vi "Read INI String.vi"(6 "Force Default Session?(F)":bool, 8 "error in (no error)":errorcluster, 9 "Default":string, 10 "Variable":T1, 11 "CSM-Static-Variable-Manager in":refnum<class "CSM-Static-Variable-Manager.lvclass">) -> (0 "error out":errorcluster, 1 "Content":string, 2 "Key Found?":bool, 3 "CSM-Static-Variable-Manager out":refnum<class "CSM-Static-Variable-Manager.lvclass">, 5 "Section Name":string)   [LabVIEW 2017, in "INI-Static-Variable-Support.lvlib" / "CSM-Static-Variable-Manager.lvclass"]
uses:
  CSM-Static-Variable-Manager.lvclass
  _Def-Ini-Variable.ctl
  CSM-Static-Variable-Manager.lvclass/CSM-Static-Variable-Manager.ctl
  INI-Static-Variable-Support.lvlib
  LabVIEW-Config/LabVIEW-Config.lvlib
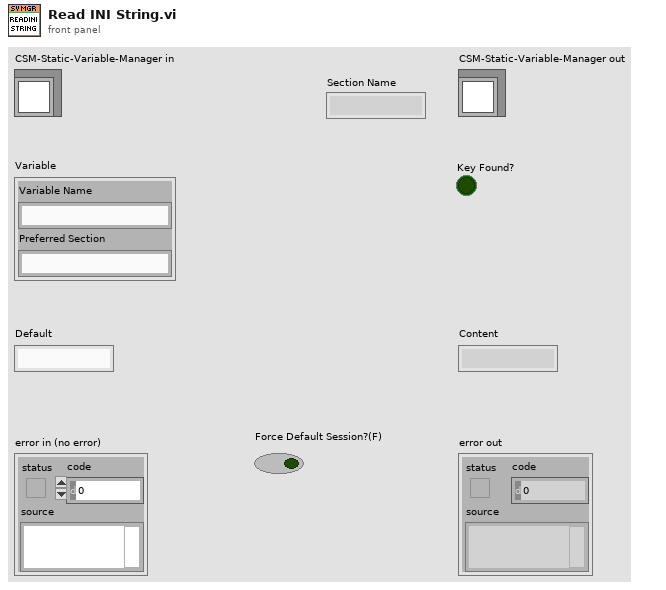
[diagram p1: front panel]
types:
  T1 = typedef "INI-Static-Variable-Support.lvlib/_Def-Ini-Variable.ctl" = cluster{"Variable Name":string, "Preferred Section":string}
  T2 = typedef "LabVIEW-Config.lvlib/Config.ctl" = cluster{"Path":path, "Lines":string[], "Tokens":T3[], "Modified?":bool}
  T3 = typedef "LabVIEW-Config.lvlib/LineToken.ctl" = enum8{"comment", "section", "key", "more"}
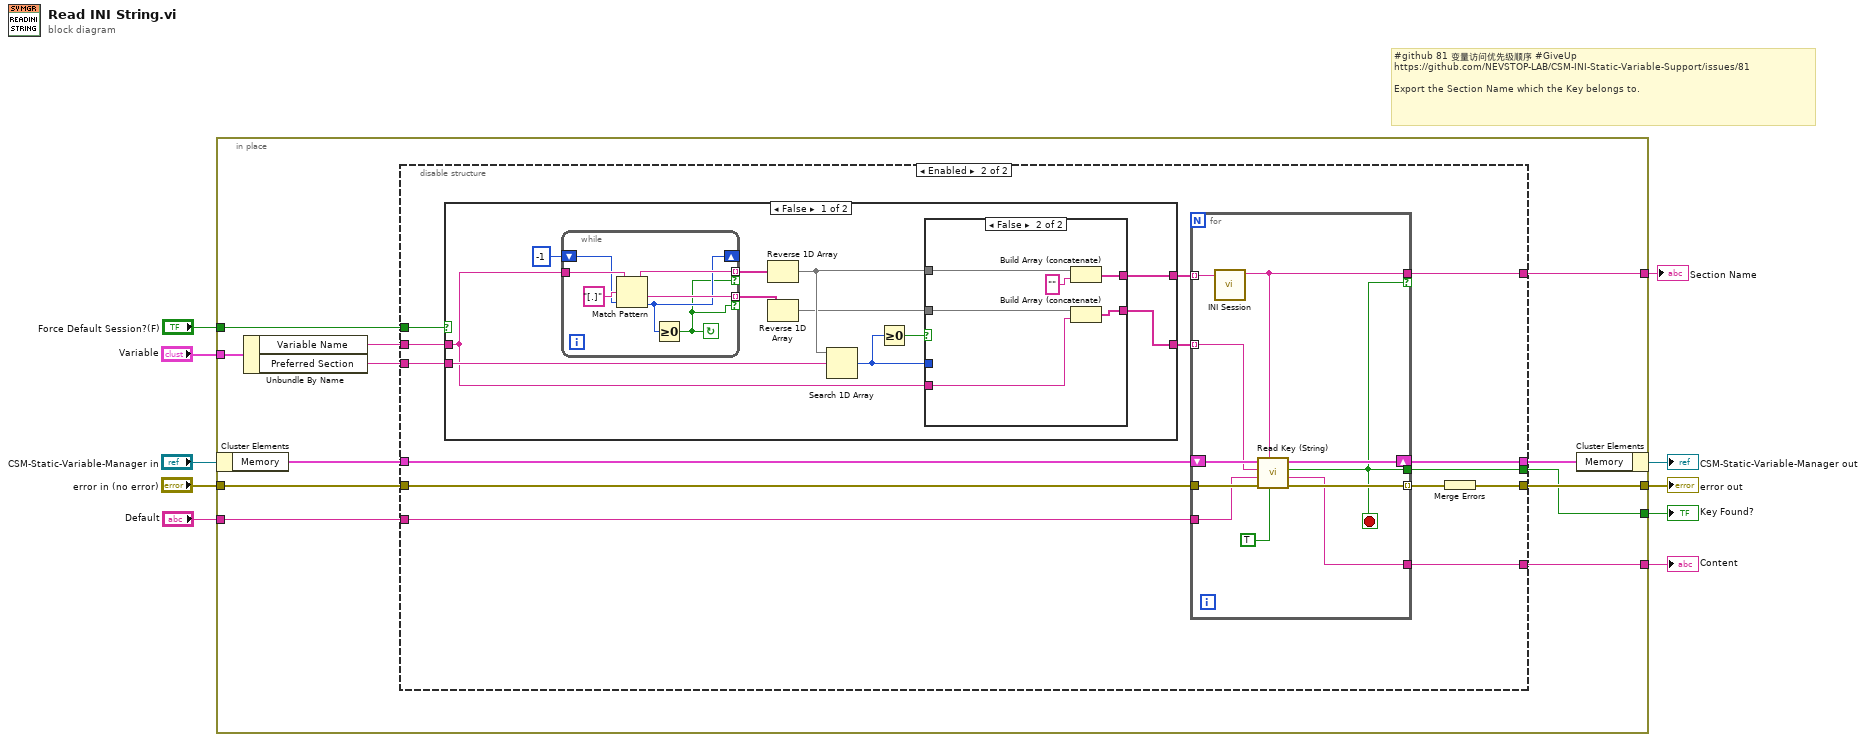
[diagram p0: block diagram]
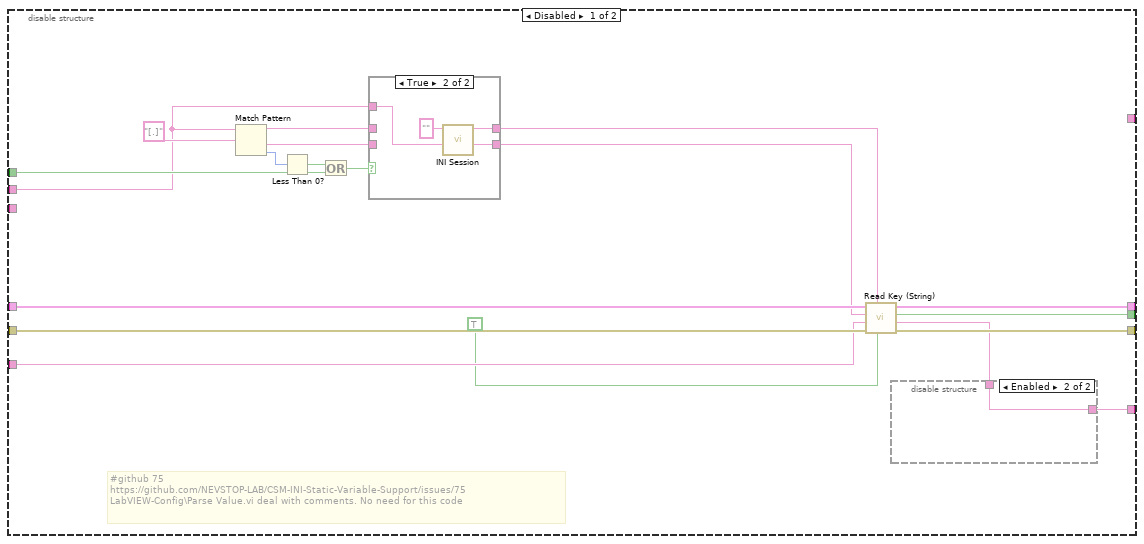
[diagram p2: hidden frame]
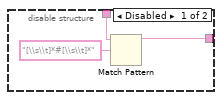
[diagram p3: hidden frame]
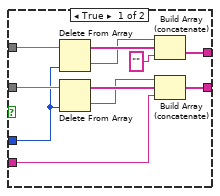
[diagram p5: hidden frame]
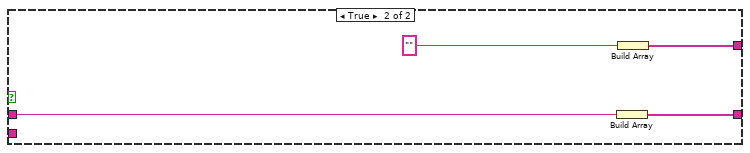
[diagram p6: hidden frame]
diagram:
  # "#github 81 变量访问优先级顺序 #GiveUp\nhttps://github.com/NEVSTOP-LAB/CSM-INI-Static-Variable-Support/issues/81\n\nExport the Section Name which the Key belongs to."
  n1 = in-place {
    in-place-border: "error in (no error)" -> [w20]
    in-place-border: [w19] -> w7
    in-place-border: [w18] -> w6
    in-place-border: "Variable" -> [w16]
    in-place-border: "Force Default Session?(F)" -> [w17]
    in-place-border: [w14] -> w3
    in-place-border: "Default" -> [w15]
    in-place-border: [w11] -> w1
    n2 = in-place-cluster #1("CSM-Static-Variable-Manager in") -> ("Memory"=w22:T2)
    n3 = Unbundle By Name(w16) -> ("Variable Name"=w13:string, "Preferred Section"=w12:string)
    n4 = disable-structure shown="Enabled" {
      disable-tunnel: w22 -> [w41 w64]
      disable-tunnel: [w40 w63] -> w21
      disable-tunnel: w20 -> [w39 w62]
      disable-tunnel: [w38 w53] -> w19
      disable-tunnel: [w37 w60] -> w18
      disable-tunnel: w17 -> [w33 w59]
      disable-tunnel: w15 -> [w27 w56]
      disable-tunnel: [w25 w55] -> w14
      disable-tunnel: w13 -> [w23 w54]
      disable-tunnel: w12 -> [_ w52]
      disable-tunnel: [_ w51] -> w11
      frame Disabled {
        # "#github 75\nhttps://github.com/NEVSTOP-LAB/CSM-INI-Static-Variable-Support/issues/75 \nLabVIEW-Config\\Parse Value.vi deal with comments. No need for this code"
        n5 = Match Pattern(string=w23, regular expression="[.]") -> (before substring=w30:string, after substring=w29:string, offset past match=w35:i32)  [unwired: 1 in, 1 out]
        n6 = Less Than 0?(x=w35) -> (x < 0?=w34:bool)
        n7 = Or(x=w34, y=w33) -> (x .or. y?=w32:bool)
        n8 = case shown="True" w32 {
          tunnel: [w47 w50] -> w31
          tunnel: w30 -> [w47 _]
          tunnel: w23 -> [_ w49]
          tunnel: w29 -> [w46 _]
          tunnel: [w46 w49] -> w28
          frame False {
          }
          frame True {
            n9 = call "INI Session.vi"("Section Name(\"\" as Default)"="" ("Section Name(\"\" as Default)")) -> ("App.Name"=w50:string)  [unwired: 10 in]
          }
        }
        n10 = call "Read Key (String).vi"("Read Raw String? (F)"=TRUE, "Section Name"=w31, "error in (no error)"=w39, "Default"=w27, "Key Name"=w28, "Config in"=w41) -> ("error out"=w38:errorcluster, "Value"=w26:string, "Key Found?"=w37:bool, "Config out"=w40:T2)  [unwired: 2 in]
        n11 = disable-structure shown="Enabled" {
          disable-tunnel: w26 -> [w44 w45]
          disable-tunnel: [w42 w45] -> w25
          frame Disabled {
            n12 = Match Pattern(string=w44, regular expression="[\\s\\t]*#[\\s\\t]*") -> (before substring=w42:string)  [unwired: 1 in, 3 out]
          }
          frame Enabled {
          }
        }
      }
      frame Enabled {
        n13 = case shown="False" w59 {
          tunnel: [w79 w113] -> w58
          tunnel: [w78 w112] -> w57
          tunnel: w54 -> [w80 w114]
          tunnel: w52 -> [w83 _]
          frame False {
            n14 = while {
              tunnel: [w108] -> w84 mode=indexing if=w104
              tunnel: [w107] -> w85 mode=indexing if=w104
              shift-right: [w105] -> _
              shift-left: -1 ("offset (0)") -> [w106]
              tunnel: w80 -> [w110]
              stop <- w104 continue-if-true
              n15 = Match Pattern(string=w110, regular expression="[.]", offset (0)=w106) -> (before substring=w108:string, after substring=w107:string, offset past match=w105:i32)  [unwired: 1 out]
              n16 = Greater Or Equal To 0?(x=w105) -> (x >= 0?=w104:bool)
            }
            n17 = Reverse 1D Array(array=w84) -> (reversed array=w82:string[])
            n18 = Reverse 1D Array(array=w85) -> (reversed array=w81:string[])
            n19 = Search 1D Array(1D array=w82, element=w83) -> (index of element=w77:i32)  [unwired: 1 in]
            n20 = Greater Or Equal To 0?(x=w77) -> (x >= 0?=w76:bool)
            n21 = case shown="False" w76 {
              tunnel: w82 -> [w97 w103]
              tunnel: w81 -> [w96 w102]
              tunnel: w80 -> [w91 w101]
              tunnel: [w89 w99] -> w79
              tunnel: [w88 w98] -> w78
              tunnel: w77 -> [w87 _]
              frame True {
                n22 = Delete From Array(array=w97, index=w87) -> (deleted portion=w92:string, array with subset deleted=w95:string[])  [unwired: 1 in]
                n23 = Delete From Array(array=w96, index=w87) -> (deleted portion=w93:string, array with subset deleted=w94:string[])  [unwired: 1 in]
                n24 = Build Array (concatenate)(w92, w95, "" ("deleted portion")) -> (w89:string[])
                n25 = Build Array (concatenate)(w93, w94, w91) -> (w88:string[])
              }
              frame False {
                n26 = Build Array (concatenate)(w103, "" ("deleted portion")) -> (w99:string[])
                n27 = Build Array (concatenate)(w102, w101) -> (w98:string[])
              }
            }
          }
          frame True {
            n28 = Build Array(w114) -> (w112:string[])
            n29 = Build Array("" ("Section Name(\"\" as Default)")) -> (w113:string[])
          }
        }
        n30 = for {
          tunnel: [w65] -> w60
          tunnel: w58 -> [w67] mode=indexing
          tunnel: w57 -> [w71] mode=indexing
          shift-right: [w74] -> w63
          shift-left: w64 -> [w75]
          tunnel: w56 -> [w70]
          tunnel: [w69] -> w55
          tunnel: w62 -> [w73]
          tunnel: [w72] -> w61 mode=indexing
          tunnel: [w66] -> w51 if=w65
          stop <- w65 stop-if-true
          n31 = call "INI Session.vi"("Section Name(\"\" as Default)"=w67) -> ("App.Name"=w66:string)  [unwired: 10 in]
          n32 = call "Read Key (String).vi"("Read Raw String? (F)"=TRUE, "Section Name"=w66, "error in (no error)"=w73, "Default"=w70, "Key Name"=w71, "Config in"=w75) -> ("error out"=w72:errorcluster, "Value"=w69:string, "Key Found?"=w65:bool, "Config out"=w74:T2)  [unwired: 2 in]
        }
        n33 = Merge Errors(w61) -> (w53:errorcluster)
      }
    }
    n34 = in-place-cluster #1("Memory"=w21) -> (→"CSM-Static-Variable-Manager out":refnum<class "CSM-Static-Variable-Manager.lvclass">)
  }
  "error out" <- w7
  "Key Found?" <- w6
  "Content" <- w3
  "Section Name" <- w1
